vi "V to Humidity converter.vi"(1 "Waveform":dbl) -> (0 "Numeric":dbl)   [LabVIEW 2022 SP3]
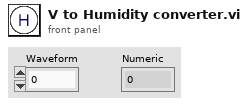
[diagram p1: front panel]
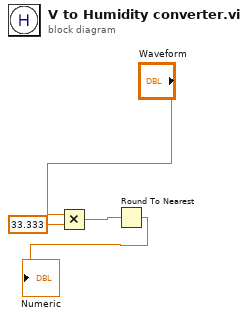
[diagram p0: block diagram]
diagram:
  n1 = Multiply(x="Waveform", y=33.333) -> (x*y=w3:dbl)
  n2 = Round To Nearest(number=w3) -> (nearest integer value=→"Numeric":dbl)
